vi "TestModbus.vi"() -> ()   [LabVIEW 2024]
uses:
  <vilib>/NI/Modbus Library/API/Wrapper/Create TCP Master.vi
  <vilib>/NI/Modbus Library/API/Master/Modbus Master.lvclass
  <vilib>/NI/Modbus Library/API/Wrapper/API Main.lvlib
panel:
  out "Array":sgl[][](array[numeric])
  out "16bit integer":i16[][](array[numeric])
  out "String":string[](array[string])
  in  "Read Data Type":enum16{"String", "Intiger", "DBL", "SGL"}(ring)
  out "String 2":string
  out "String":string
  out "register values 3":u16[](array[numeric])
  out "register values 2":u16[](array[numeric])
  # "UMESH 73"
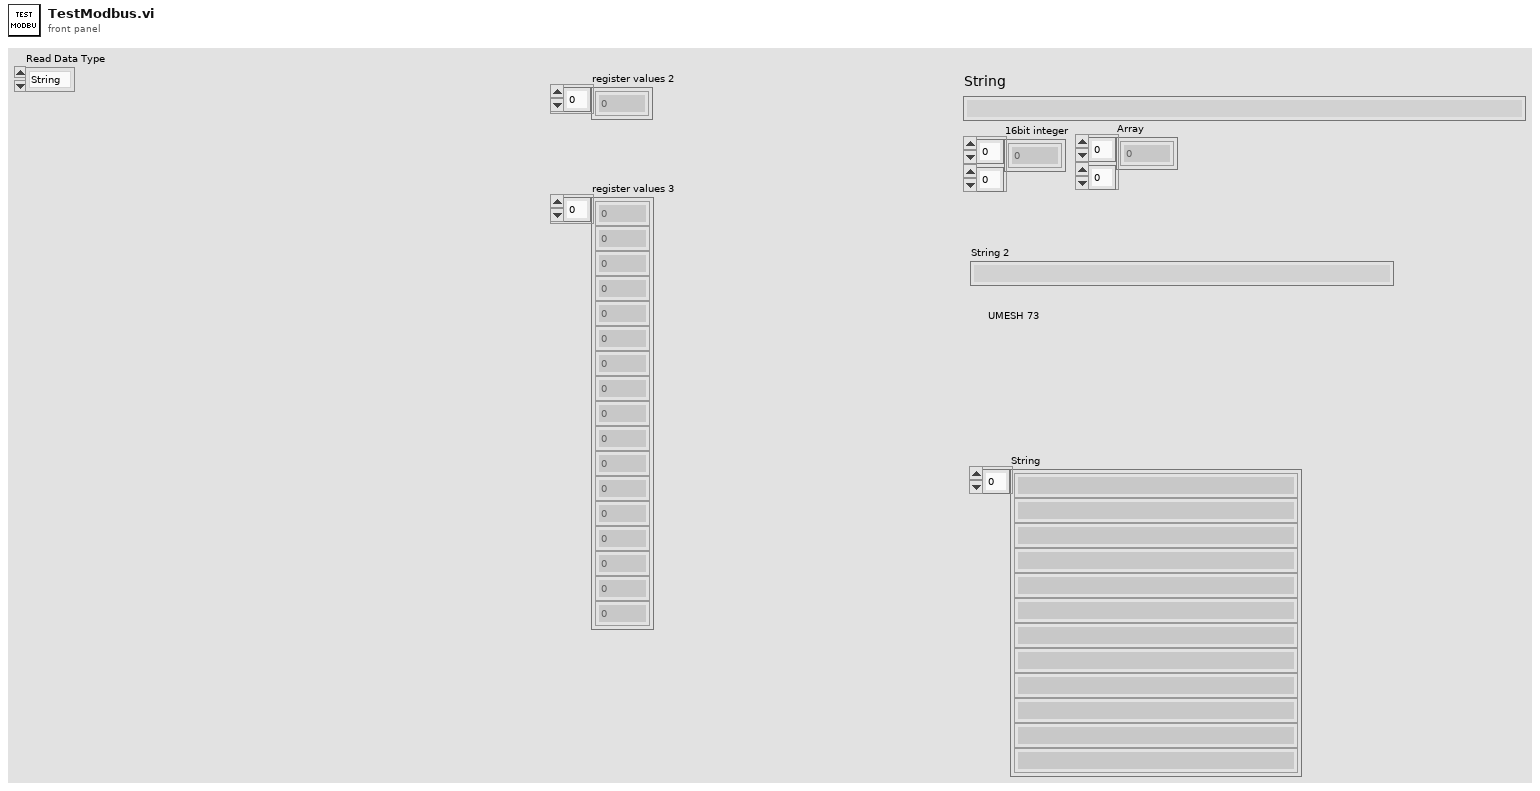
[diagram p1: front panel]
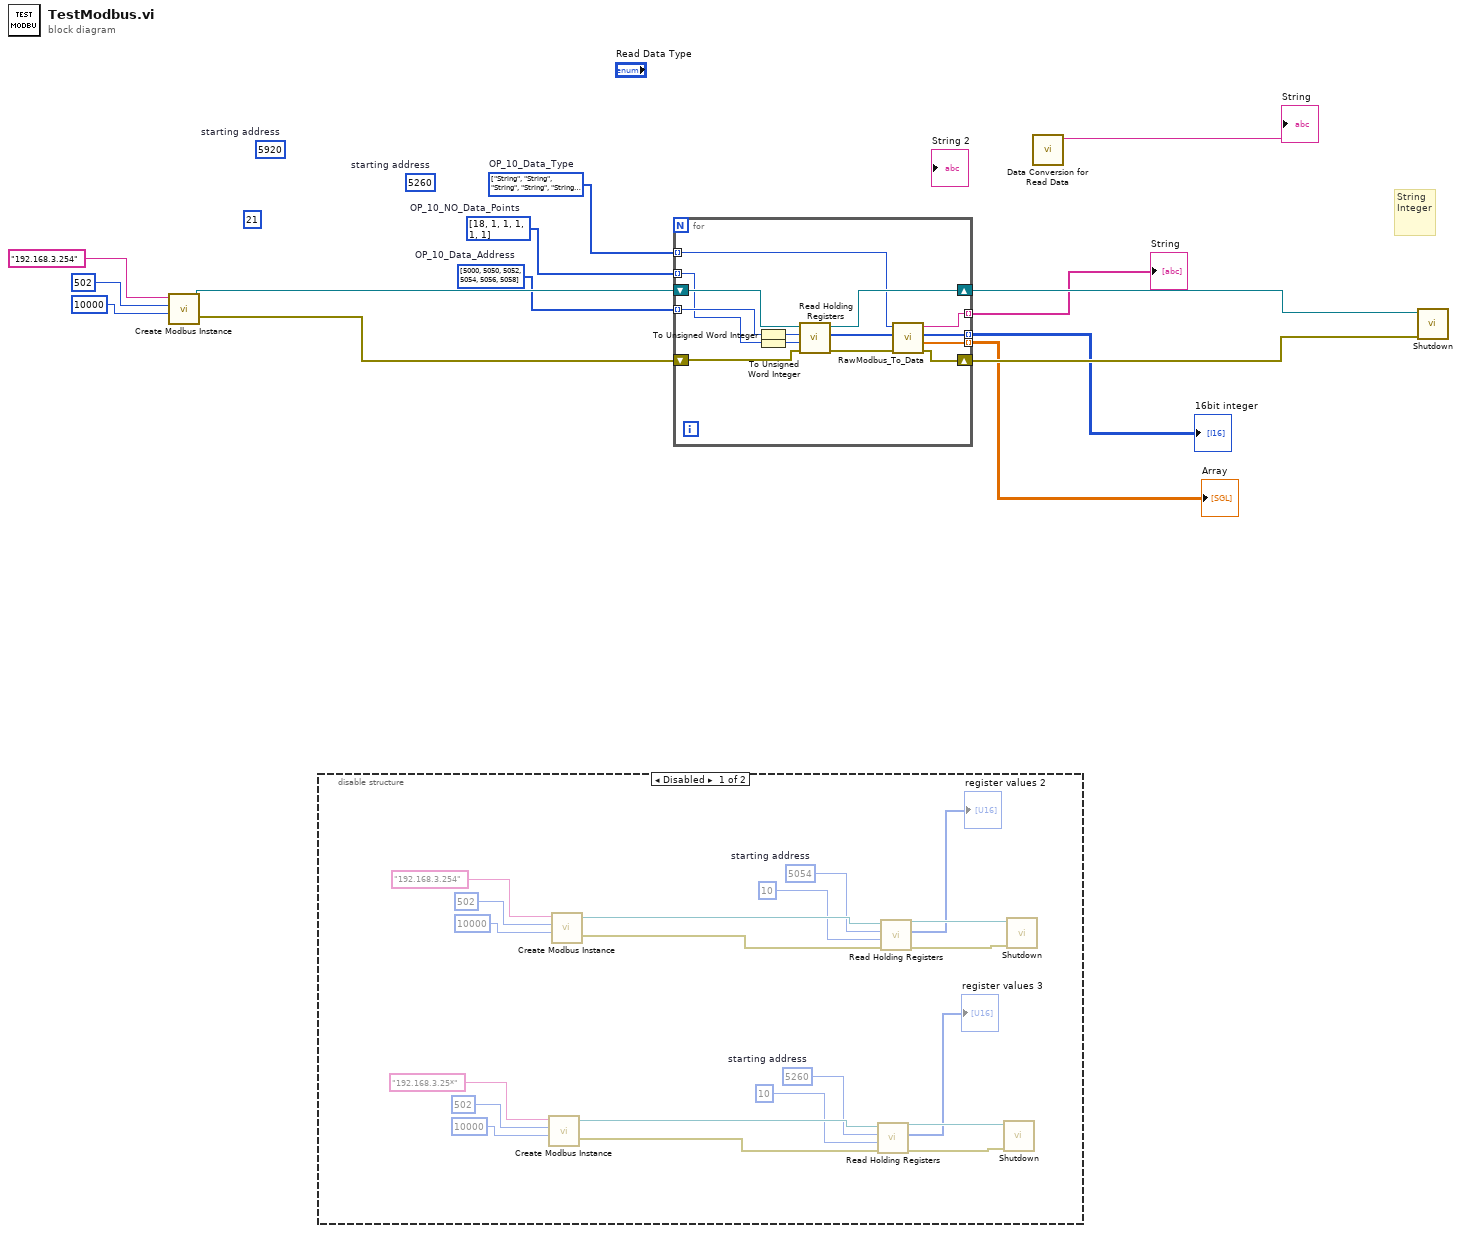
[diagram p0: block diagram]
diagram:
  w3 = i32[] [5000, 5050, 5052, 5054, 5056, 5058]  # OP_10_Data_Address
  w4 = i32[] [18, 1, 1, 1, 1, 1]  # OP_10_NO_Data_Points
  w5 = enum16{"String", "Intiger", "DBL", "SGL"}[] [enum."String", enum."String", enum."String", enum."String", enum."String", enum."String"] items=["String", "Intiger", "DBL", "SGL"]  # OP_10_Data_Type
  (unwired) u16 21 ("number of inputs")
  (unwired) u16 5920  # starting address
  (unwired) u16 5260  # starting address
  # "String\nInteger"
  n1 = call-poly <vilib>:"Create Modbus Instance.vi"("connect timeout ms"=10000, "port (502)"=u16 502, "address"="192.168.3.254") -> ("error out"=w10:errorcluster, "TCP master instance"=w11:refnum<class "Modbus Master.lvclass">)  [unwired: 7 in]
  n2 = disable-structure shown="Disabled" {
    frame Disabled {
      w19 = u16 5260  # starting address
      w29 = u16 5054  # starting address
      n3 = call-poly <vilib>:"Create Modbus Instance.vi"("connect timeout ms"=10000, "port (502)"=u16 502, "address"="192.168.3.25*") -> ("error out"=w20:errorcluster, "TCP master instance"=w21:refnum<class "Modbus Master.lvclass">)  [unwired: 7 in]
      n4 = call-poly <vilib>:"Create Modbus Instance.vi"("connect timeout ms"=10000, "port (502)"=u16 502, "address"="192.168.3.254") -> ("error out"=w30:errorcluster, "TCP master instance"=w31:refnum<class "Modbus Master.lvclass">)  [unwired: 7 in]
      n5 = call-dynamic "Read Holding Registers.vi"("error in"=w20, "number of inputs"=u16 10, "starting address"=w19, "Modbus master in"=w21) -> ("error out"=w16:errorcluster, "register values"=→"register values 3":u16[], "Modbus master out"=w17:refnum<class "Modbus Master.lvclass">)  [unwired: 5 in]
      n6 = call-dynamic "Read Holding Registers.vi"("error in"=w30, "number of inputs"=u16 10, "starting address"=w29, "Modbus master in"=w31) -> ("error out"=w26:errorcluster, "register values"=→"register values 2":u16[], "Modbus master out"=w27:refnum<class "Modbus Master.lvclass">)  [unwired: 5 in]
      n7 = call-dynamic "Shutdown.vi"("error in"=w16, "Modbus master in"=w17) -> ()  [unwired: 9 in, 1 out]
      n8 = call-dynamic "Shutdown.vi"("error in"=w26, "Modbus master in"=w27) -> ()  [unwired: 9 in, 1 out]
    }
    frame Enabled {
    }
  }
  n9 = for {
    tunnel: w3 -> [w46] mode=indexing
    shift-right: [w44] -> w9
    shift-left: w11 -> [w48]
    shift-right: [w42] -> w8
    shift-left: w10 -> [w47]
    tunnel: [w41] -> w1 mode=indexing
    tunnel: [w40] -> w6 mode=indexing
    tunnel: [w39] -> w2 mode=indexing
    tunnel: w5 -> [w37] mode=indexing
    tunnel: w4 -> [w38] mode=indexing
    n10 = To Unsigned Word Integer(number=w46) -> (unsigned 16bit integer=w36:u16)
    n11 = To Unsigned Word Integer(number=w38) -> (unsigned 16bit integer=w35:u16)
    n12 = call-dynamic "Read Holding Registers.vi"("error in"=w47, "number of inputs"=w35, "starting address"=w36, "Modbus master in"=w48) -> ("error out"=w45:errorcluster, "register values"=w43:u16[], "Modbus master out"=w44:refnum<class "Modbus Master.lvclass">)  [unwired: 5 in]
    n13 = call "RawModbus_To_Data.vi"("ErrorIn"=w45, "InpuData"=w43, "Read Data Type"=w37) -> ("ErrorOut"=w42:errorcluster, "Array"=w41:sgl[], "16bit integer"=w39:i16[], "String"=w40:string)  [unwired: 5 in]
  }
  "String" <- w6
  "16bit integer" <- w2
  "Array" <- w1
  n14 = call "Data Conversion for Read Data.vi"() -> ("String"=→"String":string)  [unwired: 8 in, 3 out]
  n15 = call-dynamic "Shutdown.vi"("error in"=w8, "Modbus master in"=w9) -> ()  [unwired: 9 in, 1 out]
